vi "SetEpsilon.vi"(7 "y?":bool, 8 "error in (no error)":errorcluster, 10 "Value in":dbl, 11 "QR Code Detector in":refnum<class "QR Code Detector.lvclass">) -> (0 "error out":errorcluster)   [LabVIEW 2020, in "feature_detection.lvlib" / "QR Code Detector.lvclass"]
uses:
  QR Code Detector.lvclass
  QR Code Detector.lvclass/QR Code Detector.ctl
  common/common.lvlib
  common/bin/gartoolkit_fd_32-1.dll
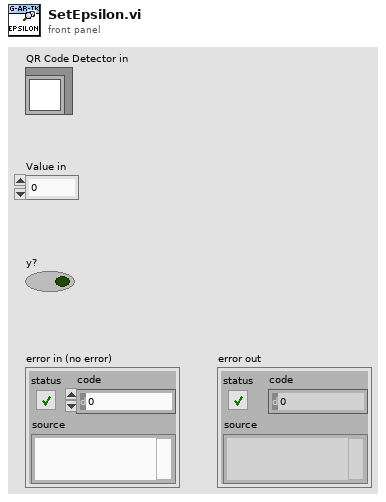
[diagram p1: front panel]
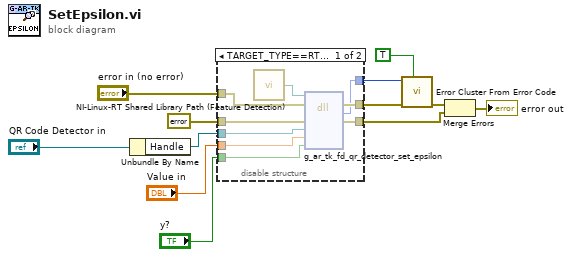
[diagram p0: block diagram]
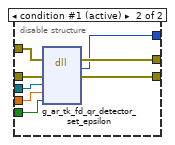
[diagram p2: hidden frame]
diagram:
  n1 = Unbundle By Name("QR Code Detector in") -> ("Handle"=w8:refnum<data-value>)
  n2 = disable-structure shown="TARGET_TYPE==RT&&OS==Linux" {
    disable-tunnel: "error in (no error)" -> [w21 w29]
    disable-tunnel: errorcluster {"status"=FALSE, "code"=0, "source"=""} ("error constant") -> [w20 w28]
    disable-tunnel: w8 -> [w19 w27]
    disable-tunnel: "Value in" -> [w18 w26]
    disable-tunnel: "y?" -> [w17 w25]
    disable-tunnel: [w16 w24] -> w5
    disable-tunnel: [w15 w23] -> w4
    disable-tunnel: [w13 w22] -> w1
    frame condition #0 {
      n3 = call "NI-Linux-RT Shared Library Path (Feature Detection).vi"() -> ("Path"=w14:path)
      n4 = dll-call lib="?" fn="g_ar_tk_fd_qr_detector_set_epsilon" ("g_ar_toolkit.*.*:g_ar_tk_capture_context_create")(path in=w14, error in=w21, "error_cluster"=w20, "Detector_EDVR"=w19, "Value"=w18, "set y?"=w17) -> (error out=w16:errorcluster, w15:i32, "error_cluster"=w13:errorcluster)  [unwired: 4 in, 1 out]
    }
    frame condition #1 (active) {
      n5 = dll-call lib="C:/serenial/lib/g-augmented-reality-toolkit/LabVIEW/common/bin/gartoolkit_fd_*-1.*" fn="g_ar_tk_fd_qr_detector_set_epsilon" ("g_ar_toolkit.*.*:g_ar_tk_capture_context_create")(error in=w29, "error_cluster"=w28, "Detector_EDVR"=w27, "Value"=w26, "set y?"=w25) -> (error out=w24:errorcluster, w23:i32, "error_cluster"=w22:errorcluster)  [unwired: 5 in, 1 out]
    }
  }
  n6 = call <vilib>:"Error Cluster From Error Code.vi"("show call chain? (False)"=TRUE, "error in (no error)"=w5, "error code (0)"=w4) -> ("error out"=w12:errorcluster)  [unwired: 6 in]
  n7 = Merge Errors(w12, w1) -> (→"error out":errorcluster)
